vi "SW_Blend_colors.vi"(8 "Background color":u32, 9 "Overlay color":u32, 10 "Blend factor":dbl, 11 "1 - Blend factor":dbl) -> (3 "Resulting color":u32)   [LabVIEW 2018, in "Tracker.lvlib"]
uses:
  Tracker.lvlib
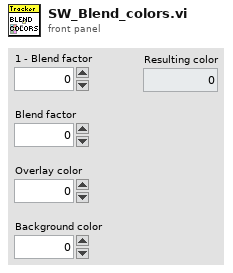
[diagram p1: front panel]
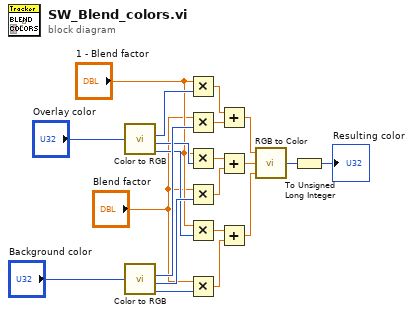
[diagram p0: block diagram]
diagram:
  n1 = call <vilib>:"Color to RGB.vi"("Color"="Overlay color") -> ("R"=w18:u8, "G"=w12:u8, "B"=w8:u8)  [unwired: 1 out]
  n2 = call <vilib>:"Color to RGB.vi"("Color"="Background color") -> ("R"=w17:u8, "G"=w11:u8, "B"=w7:u8)  [unwired: 1 out]
  n3 = Multiply(x="1 - Blend factor", y=w18) -> (x*y=w16:dbl)
  n4 = Multiply(x="Blend factor", y=w17) -> (x*y=w15:dbl)
  n5 = Multiply(x="1 - Blend factor", y=w12) -> (x*y=w13:dbl)
  n6 = Multiply(x="Blend factor", y=w11) -> (x*y=w14:dbl)
  n7 = Multiply(x="1 - Blend factor", y=w8) -> (x*y=w10:dbl)
  n8 = Multiply(x="Blend factor", y=w7) -> (x*y=w9:dbl)
  n9 = Add(x=w16, y=w15) -> (x+y=w4:dbl)
  n10 = Add(x=w13, y=w14) -> (x+y=w3:dbl)
  n11 = Add(x=w10, y=w9) -> (x+y=w2:dbl)
  n12 = call <vilib>:"RGB to Color.vi"("B"=w2, "G"=w3, "R"=w4) -> ("Color"=w1:u32)
  n13 = To Unsigned Long Integer(number=w1) -> (unsigned 32bit integer=→"Resulting color":u32)
